vi "Draw NTeeth Picture.vi"(5 "CycleAngle?":T1 caption="FPGA Simulation Angle Reference", 6 "TDC Configuration":T2(ring), 7 "Tooth/Gap Duty Cycle":dbl=50.0, 8 "error in (no error)":errorcluster, 9 "Location of Missing Teeth After TDC":dbl=300.0, 10 "Number of Missing Teeth":u8=2, 11 "Number of Teeth":u8=60) -> (0 "error out":errorcluster, 3 "N Teeth M Missing View":picture)   [LabVIEW 2011, in "Engine Sim System Explorer.lvlib"]
uses:
  Engine Sim System Explorer.lvlib
  TypeDefs/AngleReference.ctl
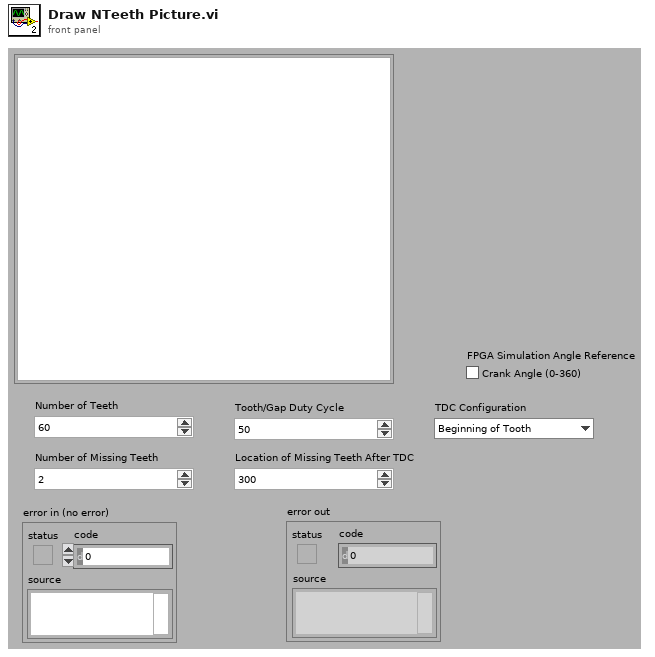
[diagram p1: front panel]
types:
  T1 = typedef "Engine Sim System Explorer.lvlib/AngleReference.ctl" = bool
  T2 = enum16{"Beginning of Tooth", "Middle of Tooth", "Beginning of Gap", "Middle of Gap"}
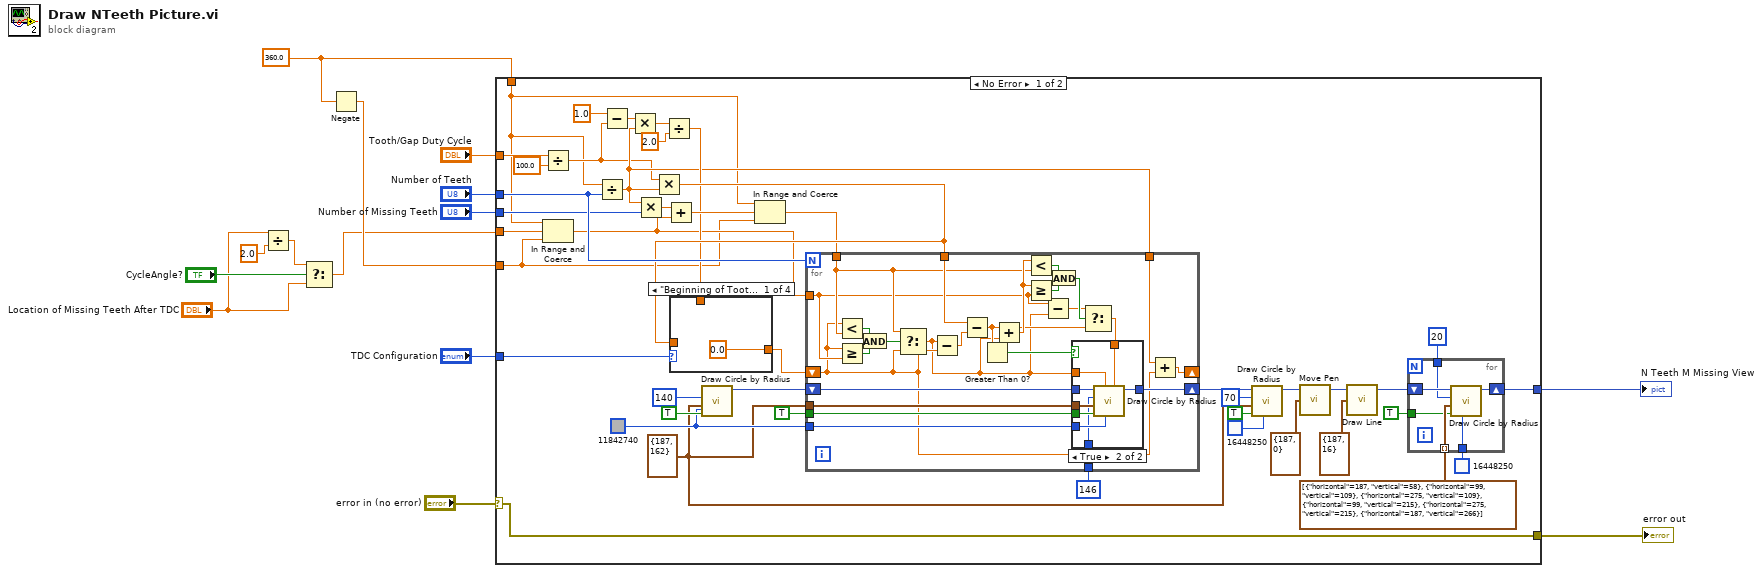
[diagram p0: block diagram]
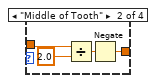
[diagram p2: hidden frame]
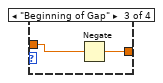
[diagram p3: hidden frame]
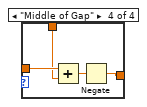
[diagram p4: hidden frame]
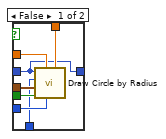
[diagram p5: hidden frame]
diagram:
  w6 = 360.0 ("upper limit")
  n1 = Divide(x="Location of Missing Teeth After TDC", y=2.0) -> (x/y=w2:dbl)
  n2 = Select(t=w2, s="CycleAngle?", f="Location of Missing Teeth After TDC") -> (s? t:f=w4:dbl)
  n3 = Negate(x=w6) -> (-x=w7:dbl)
  n4 = case shown="No Error" "error in (no error)" {
    selector: "error in (no error)" -> [w19 w115]
    tunnel: "Number of Teeth" -> [w53 _]
    tunnel: "Number of Missing Teeth" -> [w52 _]
    tunnel: w4 -> [w50 _]
    tunnel: "Tooth/Gap Duty Cycle" -> [w48 _]
    tunnel: [w32 _] -> w11
    tunnel: "TDC Configuration" -> [w31 _]
    tunnel: [w19 w115] -> w8
    tunnel: w6 -> [w16 _]
    tunnel: w7 -> [w15 _]
    frame No Error {
      w46 = u32 11842740 ("color(black)")
      w29 = cluster{"horizontal":i16, "vertical":i16} {"horizontal"=187, "vertical"=162} ("pixel center")
      n5 = Divide(x=w48, y=100.0) -> (x/y=w20:dbl)
      n6 = In Range and Coerce(upper limit=w16, x=w50, lower limit=w15) -> (coerced(x)=w18:dbl)  [unwired: 1 out]
      n7 = Divide(x=w16, y=w53) -> (x/y=w21:dbl)
      n8 = Subtract(x=1.0, y=w20) -> (x-y=w25:dbl)
      n9 = Multiply(x=w25, y=w21) -> (x*y=w24:dbl)
      n10 = Multiply(x=w21, y=w52) -> (x*y=w51:dbl)
      n11 = Multiply(x=w20, y=w21) -> (x*y=w27:dbl)
      n12 = Divide(x=w24, y=2.0) -> (x/y=w22:dbl)
      n13 = Add(x=w51, y=w18) -> (x+y=w49:dbl)
      n14 = case shown="\"Beginning of Tooth\", Default" w31 {
        tunnel: [0.0 w59 w63 w65] -> w30
        tunnel: w27 -> [_ w61 w64 w68]
        tunnel: w22 -> [_ _ _ w67]
        frame "Beginning of Tooth", Default {
        }
        frame "Middle of Tooth" {
          n15 = Divide(x=w61, y=2.0) -> (x/y=w62:dbl)
          n16 = Negate(x=w62) -> (-x=w59:dbl)
        }
        frame "Beginning of Gap" {
          n17 = Negate(x=w64) -> (-x=w63:dbl)
        }
        frame "Middle of Gap" {
          n18 = Add(x=w68, y=w67) -> (x+y=w66:dbl)
          n19 = Negate(x=w66) -> (-x=w65:dbl)
        }
      }
      n20 = call <vilib>:"Draw Circle by Radius.vi"("color(black)"=w46, "fill?(F)"=TRUE, "pixel center"=w29, "radius"=i16 140) -> ("new picture"=w56:picture)  [unwired: 7 in]
      n21 = In Range and Coerce(upper limit=w16, x=w49, lower limit=w15) -> (coerced(x)=w17:dbl)  [unwired: 1 out]
      n22 = for {
        N: w53 -> [_]
        tunnel: TRUE ("fill?(F)") -> [w97]
        tunnel: w29 -> [w96]
        shift-right: [w98] -> w45
        shift-left: w56 -> [w99]
        shift-right: [w95] -> _
        shift-left: w30 -> [w77]
        tunnel: w27 -> [w88]
        tunnel: w21 -> [w94]
        tunnel: w18 -> [w79]
        tunnel: w17 -> [w80]
        tunnel: w46 -> [w90]
        tunnel: i16 146 ("radius") -> [w89]
        n23 = Less?(x=w77, y=w80) -> (x < y?=w93:bool)
        n24 = Greater Or Equal?(x=w77, y=w79) -> (x >= y?=w92:bool)
        n25 = And(x=w93, y=w92) -> (x .and. y?=w91:bool)
        n26 = Select(t=w80, s=w91, f=w77) -> (s? t:f=w75:dbl)
        n27 = Subtract(x=w75, y=w77) -> (x-y=w87:dbl)
        n28 = Subtract(x=w88, y=w87) -> (x-y=w78:dbl)
        n29 = Greater Than 0?(x=w78) -> (x > 0?=w86:bool)
        n30 = Add(x=w78, y=w75) -> (x+y=w81:dbl)
        n31 = Less?(x=w81, y=w80) -> (x < y?=w84:bool)
        n32 = Greater Or Equal?(x=w81, y=w79) -> (x >= y?=w83:bool)
        n33 = Subtract(x=w79, y=w75) -> (x-y=w76:dbl)
        n34 = And(x=w84, y=w83) -> (x .and. y?=w82:bool)
        n35 = Select(t=w76, s=w82, f=w78) -> (s? t:f=w85:dbl)
        n36 = case shown="True" w86 {
          tunnel: w99 -> [w101 w114]
          tunnel: [w101 w113] -> w98
          tunnel: w97 -> [w106 w112]
          tunnel: w96 -> [w105 w111]
          tunnel: w85 -> [w104 w110]
          tunnel: w75 -> [w103 w109]
          tunnel: w90 -> [w102 w108]
          tunnel: w89 -> [w100 w107]
          frame False {
            n37 = call <vilib>:"Draw Circle by Radius.vi"("arc size(360)"=w104, "color(black)"=w102, "start angle(0)"=w103, "fill?(F)"=w106, "pixel center"=w105, "radius"=w100, "picture"=w101) -> ()  [unwired: 4 in, 1 out]
          }
          frame True {
            n38 = call <vilib>:"Draw Circle by Radius.vi"("arc size(360)"=w110, "color(black)"=w108, "start angle(0)"=w109, "fill?(F)"=w112, "pixel center"=w111, "radius"=w107, "picture"=w114) -> ("new picture"=w113:picture)  [unwired: 4 in]
          }
        }
        n39 = Add(x=w94, y=w77) -> (x+y=w95:dbl)
      }
      n40 = call <vilib>:"Draw Circle by Radius.vi"("color(black)"=u32 16448250, "fill?(F)"=TRUE, "pixel center"=w29, "radius"=i16 70, "picture"=w45) -> ("new picture"=w44:picture)  [unwired: 6 in]
      n41 = call <vilib>:"Move Pen.vi"("new position"=cluster{"x":i16, "y":i16} {"x"=187, "y"=0} ("end point"), "picture"=w44) -> ("new picture"=w39:picture)  [unwired: 3 in]
      n42 = call <vilib>:"Draw Line.vi"("picture"=w39, "end point"=cluster{"x":i16, "y":i16} {"x"=187, "y"=16}) -> ("new picture"=w37:picture)  [unwired: 7 in]
      n43 = for {
        shift-right: [w73] -> w32
        shift-left: w37 -> [w74]
        tunnel: i16 20 ("radius") -> [w72]
        tunnel: cluster{"horizontal":i16, "vertical":i16}[] [{"horizontal"=187, "vertical"=58}, {"horizontal"=99, "vertical"=109}, {"horizontal"=275, "vertical"=109}, {"horizontal"=99, "vertical"=215}, {"horizontal"=275, "vertical"=215}, {"horizontal"=187, "vertical"=266}] -> [w71] mode=indexing
        tunnel: TRUE ("fill?(F)") -> [w70]
        tunnel: u32 16448250 ("color(black)") -> [w69]
        n44 = call <vilib>:"Draw Circle by Radius.vi"("color(black)"=w69, "fill?(F)"=w70, "pixel center"=w71, "radius"=w72, "picture"=w74) -> ("new picture"=w73:picture)  [unwired: 6 in]
      }
    }
    frame Error {
    }
  }
  "N Teeth M Missing View" <- w11
  "error out" <- w8
